vi "MultiPAS-III.vi"() -> ()   [LabVIEW 2011]
uses:
  <vilib>/Analysis/4window.llb/windowTd.ctl
  sub/QMH/QMH Add Message to Queue (Single Element).vi
  sub/QMH/QMH Add Message to Queue (Array).vi
  sub/absCalcPlot_III.vi
  <vilib>/Utility/file.llb/Write To Spreadsheet File (string).vi
  <vilib>/measure/maspectr.llb/FFT Spectrum (Mag-Phase) for 1 Chan.vi
  sub/fftGetMags.vi
  sub/rollingAverage_III.vi
  sub/micUnbundle_III.vi
  <vilib>/Instr/_visa.llb/VISA Configure Serial Port (Instr).vi
  sub/pdNormalize_III.vi
  <vilib>/measure/NI_MAPro.lvlib
  <vilib>/Analysis/NI_AALPro.lvlib
panel:
  out "pd ts (raw)":T1
  out "PAS Save":bool caption="Overtemp"
  in  "Data 2":i32[][](array[numeric])=[[-16374, -7248, 2543, 12030, 20279, 26487, 30037, 30583, 28073, 22744, 15131, 5976, -3818, -13288, -21504, -27663, -31155, -31636, -29064, -23686, -16036, -6862, 2936, 12388, 20571, 26684, 30122, 30546, 27911, 22483, 14793, 5595, -4207, -13644, -21795, -27855, -31232, -31591, -28898, -23423, -15695, -6476, 3323, 12743, 20858, 26873, 30194, 30492, 27744, 22213, 14447, 5207, -4597, -14002, -22082, -28044, -31304, -31540, -28731, -23149, -15348, -6093, 3713, 13101, 21145, 27063, 30265, 30442, 27576, 21943, 14103, 4822, -4984, -14354, -22365, -28230, -31373, -31485, -28556, -22876, -14998, -5702, 4104, 13452, 21428, 27245, 30335, 30388, 27400, 21669, 13754, 4435, -5375, -14705, -22643, -28407, -31436, -31426, -28378, -22598, -14648, -5314, 4497, 13803, 21706, 27423, 30394, 30325, 27221, 21390, 13402, 4045, -5763, -15056, -22921, -28586, -31496, -31361, -28198, -22319, -14297, -4924, 4879, 14151, 21982, 27597, 30451, 30257, 27038, 21107, 13050, 3658, -6149, -15402, -23193, -28754, -31546, -31290, -28010, -22033, -13944, -4536, 5266, 14498, 22252, 27767, 30500, 30184, 26849, 20821, 12696, 3267, -6535, -15748, -23462, -28924, -31596, -31216, -27821, -21748, -13587, -4147, 5653, 14838, 22519, 27930, 30549, 30110, 26658, 20535, 12337, 2878, -6919, -16089, -23727, -29087, -31641, -31137, -27627, -21457, -13229, -3753, 6038, 15181, 22786, 28093, 30591, 30031, 26461, 20243, 11979, 2485, -7303, -16428, -23991, -29244, -31678, -31053, -27426, -21159, -12867, -3360, 6424, 15524, 23043, 28252, 30633, 29946, 26262, 19946, 11617, 2096, -7686, -16764, -24246, -29398, -31712, -30964, -27224, -20862, -12503, -2971, 6803, 15859, 23301, 28401, 30661, 29852, 26058, 19648, 11254, 1703, -8069, -17099, -24500, -29547, -31741, -30870, -27018, -20562, -12138, -2575, 7188, 16192, 23556, 28549, 30689, 29756, 25848, 19348, 10891, 1312, -8448, -17430, -24753, -29691, -31765, -30773, -26806, -20259, -11775, -2186, 7566, 16521, 23801, 28690, 30709, 29656, 25634, 19038, 10523, 919, -8831, -17762, -24997, -29833, -31788, -30672, -26593, -19955, -11409, -1792, 7944, 16850, 24047, 28830, 30724, 29548, 25416, 18729, 10152, 523, -9212, -18092, -25245, -29969, -31805, -30566, -26375, -19647, -11041, -1403, 8319, 17173, 24287, 28963, 30734, 29436, 25192, 18418, 9781, 130, -9587, -18413, -25481, -30101, -31814, -30449, -26150, -19332, -10666, -1007, 8697, 17497, 24524, 29090, 30745, 29325, 24968, 18105, 9408, -263, -9962, -18735, -25718, -30228, -31820, -30334, -25921, -19016, -10296, -618, 9072, 17814, 24756, 29213, 30746, 29202, 24738, 17787, 9036, -657, -10338, -19058, -25951, -30350, -31818, -30214, -25690, -18699, -9922, -224, 9442, 18128, 24984, 29330, 30738, 29078, 24502, 17466, 8658, -1050, -10710, -19371, -26178, -30467, -31814, -30088, -25458, -18382, -9550, 167, 9812, 18440, 25206, 29443, 30732, 28947, 24264, 17143, 8281, -1445, -11083, -19685, -26404, -30581, -31807, -29959, -25221, -18059, -9175, 556, 10178, 18750, 25426, 29548, 30718, 28809, 24018, 16812, 7901, -1842, -11457, -19996, -26624, -30690, -31795, -29824, -24980, -17733, -8799, 950, 10549, 19058, 25643, 29655, 30700, 28673, 23773, 16484, 7523, -2235, -11824, -20304, -26840, -30793, -31772, -29682, -24731, -17402, -8415, 1341, 10916, 19363, 25856, 29755, 30677, 28528, 23522, 16151, 7141, -2626, -12191, -20607, -27051, -30891, -31746, -29536, -24481, -17070, -8035, 1733, 11280, 19664, 26064, 29851, 30648, 28381, 23272, 15818, 6762, -3019, -12555, -20906, -27258, -30984, -31717, -29391, -24226, -16736, -7655, 2128, 11641, 19962, 26270, 29940, 30615, 28229, 23013, 15483, 6376, -3409, -12914, -21204, -27459, -31071, -31684, -29236, -23967, -16398, -7271, 2515, 12005, 20258, 26468, 30024, 30577, 28072, 22753, 15143, 5990, -3802, -13276, -21497, -27660, -31157, -31643, -29076, -23707, -16058, -6886, 2908, 12363, 20550, 26666, 30107, 30536, 27914, 22489, 14805, 5607, -4192, -13633, -21787, -27849, -31230, -31597, -28911, -23438, -15716, -6501, 3298, 12719, 20839, 26858, 30182, 30488, 27744, 22223, 14459, 5225, -4579, -13988, -22071, -28040, -31304, -31549, -28743, -23167, -15368, -6113, 3693, 13076, 21126, 27047, 30255, 30438, 27576, 21950, 14113, 4837, -4971, -14340, -22354, -28224, -31375, -31494, -28570, -22895, -15022, -5725, 4080, 13430, 21408, 27230, 30324, 30384, 27402, 21676, 13766, 4449, -5360, -14694, -22636, -28409, -31440, -31436, -28397, -22617, -14674, -5338, 4467, 13781, 21686, 27408, 30385, 30320, 27224, 21398, 13418, 4062, -5748, -15044, -22913, -28584, -31498, -31368, -28212, -22339, -14321, -4948, 4856, 14131, 21963, 27583, 30440, 30254, 27042, 21118, 13062, 3669, -6137, -15390, -23183, -28751, -31551, -31297, -28024, -22049, -13962, -4556, 5245, 14476, 22235, 27754, 30497, 30186, 26857, 20834, 12710, 3283, -6519, -15733, -23453, -28921, -31600, -31226, -27837, -21765, -13610, -4168, 5628, 14820, 22502, 27918, 30540, 30109, 26664, 20544, 12354, 2891, -6906, -16074, -23719, -29085, -31646, -31148, -27642, -21475, -13251, -3777, 6014, 15160, 22765, 28078, 30583, 30027, 26468, 20251, 11994, 2501, -7292, -16415, -23980, -29242, -31682, -31064, -27443, -21181, -12892, -3386, 6397, 15501, 23026, 28238, 30624, 29944, 26269, 19959, 11633, 2110, -7673, -16753, -24239, -29395, -31719, -30974, -27239, -20882, -12528, -2993, 6782, 15835, 23285, 28390, 30651, 29852, 26063, 19660, 11271, 1720, -8053, -17087, -24493, -29546, -31746, -30880, -27031, -20583, -12163, -2599, 7166, 16173, 23538, 28538, 30684, 29758, 25853, 19356, 10906, 1327, -8433, -17416, -24743, -29688, -31769, -30782, -26821, -20280, -11797, -2208, 7543, 16501, 23786, 28680, 30704, 29656, 25642, 19053, 10540, 936, -8814, -17747, -24989, -29827, -31787, -30678, -26606, -19973, -11430, -1817, 7923, 16829, 24031, 28819, 30721, 29552, 25424, 18746, 10174, 543, -9191, -18072, -25231, -29962, -31802, -30567, -26384, -19660, -11057, -1422, 8302, 17159, 24274, 28952, 30738, 29443, 25205, 18435, 9801, 150, -9568, -18401, -25472, -30095, -31811, -30457, -26163, -19349, -10687, -1031, 8679, 17481, 24511, 29082, 30742, 29327, 24979, 18121, 9431, -241, -9943, -18717, -25707, -30221, -31815, -30337, -25930, -19029, -10312, -631, 9058, 17802, 24745, 29207, 30746, 29209, 24750, 17805, 9057, -634, -10316, -19037, -25937, -30340, -31814, -30217, -25700, -18713, -9939, -240, 9429, 18117, 24976, 29328, 30740, 29088, 24519, 17486, 8682, -1027, -10688, -19352, -26164, -30458, -31810, -30091, -25465, -18390, -9561, 154, 9800, 18433, 25201, 29442, 30735, 28959, 24282, 17165, 8308, -1420, -11063, -19665, -26386, -30570, -31801, -29961, -25227, -18068, -9185, 547, 10171, 18745, 25424, 29552, 30726, 28825, 24038, 16835, 7925, -1815, -11429, -19974, -26608, -30681, -31789, -29826, -24984, -17741, -8807, 938, 10536, 19047, 25636, 29657, 30708, 28685, 23794, 16510, 7550, -2205, -11798, -20280, -26821, -30782, -31766, -29684, -24737, -17411, -8429, 1331, 10906, 19356, 25851, 29758, 30684, 28544, 23546, 16178, 7169, -2598, -12162, -20582, -27035, -30879, -31744, -29540, -24485, -17080, -8048, 1721, 11267, 19655, 26061, 29852, 30654, 28395, 23291, 15843, 6786, -2993, -12527, -20884, -27240, -30974, -31713, -29390, -24230, -16744, -7662, 2115, 11635, 19957, 26268, 29945, 30624, 28246, 23035, 15509, 6406, -3382, -12889, -21180, -27444, -31061, -31677, -29236, -23975, -16408, -7284], [-19329, -1252, 17344, 29341, 30145, 19451, 1353, -17227, -29174, -29920, -19175, -1056, 17506, 29408, 30095, 19300, 1159, -17387, -29238, -29860, -19019, -860, 17671, 29475, 30037, 19143, 960, -17553, -29307, -29809, -18866, -664, 17832, 29545, 29987, 18991, 771, -17707, -29365, -29749, -18707, -466, 17992, 29605, 29926, 18832, 570, -17873, -29434, -29694, -18556, -272, 18151, 29670, 29869, 18676, 375, -18031, -29495, -29633, -18395, -75, 18310, 29729, 29809, 18516, 175, -18194, -29561, -29579, -18238, 120, 18469, 29792, 29750, 18362, -17, -18347, -29617, -29515, -18076, 316, 18629, 29848, 29682, 18197, -218, -18510, -29679, -29456, -17921, 513, 18787, 29910, 29626, 18042, -408, -18664, -29734, -29388, -17757, 709, 18941, 29965, 29560, 17875, -609, -18823, -29791, -29326, -17600, 904, 19095, 30023, 29495, 17717, -802, -18975, -29845, -29260, -17434, 1099, 19251, 30075, 29425, 17551, -1001, -19131, -29901, -29194, -17277, 1296, 19408, 30130, 29359, 17393, -1193, -19284, -29953, -29124, -17112, 1491, 19560, 30184, 29290, 17225, -1392, -19440, -30008, -29056, -16949, 1686, 19713, 30237, 29226, 17069, -1581, -19587, -30054, -28982, -16781, 1883, 19866, 30287, 29151, 16898, -1781, -19742, -30107, -28913, -16616, 2079, 20018, 30337, 29082, 16737, -1973, -19888, -30152, -28838, -16449, 2275, 20167, 30383, 29006, 16564, -2174, -20041, -30200, -28765, -16282, 2471, 20321, 30430, 28934, 16403, -2364, -20187, -30243, -28688, -16113, 2669, 20465, 30470, 28853, 16230, -2568, -20341, -30294, -28618, -15953, 2860, 20615, 30519, 28783, 16070, -2755, -20486, -30335, -28537, -15779, 3057, 20760, 30560, 28700, 15892, -2956, -20637, -30378, -28461, -15613, 3252, 20909, 30605, 28628, 15730, -3145, -20777, -30418, -28377, -15440, 3446, 21054, 30645, 28543, 15557, -3345, -20927, -30460, -28299, -15271, 3643, 21199, 30686, 28465, 15391, -3534, -21066, -30495, -28215, -15100, 3839, 21345, 30722, 28380, 15214, -3734, -21213, -30534, -28134, -14928, 4032, 21487, 30760, 28300, 15044, -3926, -21355, -30570, -28052, -14757, 4225, 21627, 30792, 28209, 14870, -4123, -21501, -30607, -27968, -14586, 4419, 21768, 30832, 28129, 14702, -4314, -21637, -30639, -27880, -14413, 4612, 21907, 30859, 28040, 14521, -4515, -21780, -30675, -27796, -14241, 4804, 22048, 30895, 27953, 14352, -4702, -21919, -30705, -27707, -14064, 4999, 22187, 30922, 27859, 14172, -4900, -22060, -30739, -27620, -13892, 5193, 22326, 30954, 27773, 14003, -5090, -22194, -30765, -27524, -13712, 5386, 22462, 30981, 27679, 13823, -5285, -22333, -30794, -27436, -13538, 5580, 22600, 31013, 27591, 13650, -5476, -22466, -30820, -27343, -13363, 5770, 22732, 31033, 27491, 13468, -5673, -22605, -30848, -27251, -13187, 5964, 22870, 31060, 27401, 13292, -5863, -22736, -30870, -27155, -13010, 6156, 23000, 31079, 27299, 13111, -6058, -22873, -30895, -27060, -12833, 6347, 23134, 31104, 27208, 12936, -6248, -23004, -30918, -26965, -12652, 6536, 23260, 31120, 27106, 12753, -6444, -23136, -30939, -26865, -12472, 6729, 23395, 31148, 27011, 12578, -6634, -23266, -30959, -26766, -12296, 6919, 23523, 31161, 26907, 12392, -6830, -23402, -30982, -26665, -12115, 7109, 23652, 31180, 26809, 12213, -7016, -23524, -30992, -26564, -11932, 7301, 23777, 31195, 26704, 12032, -7210, -23655, -31011, -26464, -11755, 7492, 23907, 31211, 26605, 11855, -7395, -23778, -31024, -26358, -11573, 7680, 24031, 31218, 26494, 11665, -7592, -23908, -31039, -26258, -11392, 7871, 24158, 31237, 26394, 11491, -7775, -24031, -31050, -26153, -11210, 8063, 24281, 31247, 26285, 11302, -7972, -24159, -31062, -26046, -11027, 8250, 24407, 31258, 26180, 11124, -8157, -24276, -31067, -25937, -10841, 8438, 24526, 31265, 26071, 10936, -8347, -24401, -31078, -25829, -10659, 8630, 24649, 31275, 25965, 10755, -8533, -24522, -31087, -25721, -10474, 8816, 24770, 31280, 25853, 10566, -8726, -24641, -31091, -25608, -10290, 9003, 24891, 31287, 25746, 10386, -8910, -24756, -31095, -25498, -10105, 9192, 25008, 31287, 25627, 10196, -9102, -24881, -31101, -25386, -9919, 9381, 25127, 31296, 25521, 10019, -9284, -24994, -31099, -25268, -9732, 9570, 25243, 31293, 25403, 9826, -9476, -25113, -31105, -25157, -9544, 9756, 25359, 31298, 25291, 9645, -9655, -25225, -31099, -25040, -9359, 9942, 25473, 31291, 25167, 9453, -9847, -25341, -31102, -24926, -9173, 10124, 25586, 31294, 25057, 9269, -10029, -25450, -31095, -24809, -8986, 10310, 25696, 31284, 24931, 9078, -10218, -25564, -31094, -24688, -8798, 10497, 25812, 31287, 24819, 8896, -10399, -25673, -31085, -24567, -8608, 10682, 25922, 31278, 24698, 8703, -10587, -25785, -31080, -24448, -8422, 10866, 26033, 31274, 24582, 8522, -10765, -25890, -31067, -24321, -8230, 11050, 26140, 31263, 24455, 8325, -10952, -26001, -31064, -24201, -8040, 11234, 26248, 31255, 24338, 8142, -11132, -26106, -31054, -24079, -7852, 11417, 26353, 31243, 24207, 7948, -11316, -26217, -31041, -23952, -7662, 11601, 26464, 31236, 24089, 7763, -11494, -26315, -31025, -23829, -7471, 11782, 26562, 31217, 23957, 7567, -11682, -26422, -31014, -23702, -7282, 11962, 26667, 31205, 23834, 7383, -11859, -26521, -30998, -23575, -7092, 12144, 26770, 31187, 23704, 7186, -12043, -26626, -30981, -23444, -6900, 12328, 26875, 31176, 23582, 7003, -12218, -26724, -30962, -23316, -6709, 12505, 26971, 31154, 23446, 6805, -12401, -26825, -30946, -23189, -6517, 12687, 27073, 31139, 23322, 6620, -12576, -26919, -30922, -23054, -6323, 12867, 27170, 31114, 23185, 6422, -12760, -27022, -30904, -22923, -6132, 13047, 27272, 31096, 23060, 6237, -12934, -27114, -30879, -22790, -5940, 13222, 27362, 31068, 22921, 6041, -13116, -27212, -30855, -22657, -5748, 13401, 27461, 31048, 22790, 5853, -13289, -27302, -30828, -22522, -5555, 13577, 27549, 31019, 22652, 5652, -13472, -27398, -30806, -22388, -5362, 13753, 27645, 30995, 22521, 5463, -13642, -27487, -30776, -22248, -5169, 13928, 27733, 30963, 22376, 5266, -13823, -27584, -30750, -22113, -4975, 14106, 27828, 30937, 22246, 5082, -13992, -27669, -30717, -21974, -4782, 14280, 27914, 30902, 22101, 4880, -14174, -27760, -30689, -21837, -4588, 14454, 28006, 30875, 21965, 4692, -14340, -27843, -30653, -21693, -4391, 14631, 28092, 30840, 21822, 4494, -14519, -27934, -30620, -21552, -4198, 14805, 28179, 30808, 21688, 4308, -14687, -28015, -30582, -21410, -4004, 14975, 28262, 30770, 21540, 4106, -14861, -28103, -30548, -21268, -3808, 15149, 28349, 30739, 21402, 3916, -15032, -28183, -30512, -21124, -3614, 15319, 28430, 30697, 21255, 3715, -15205, -28267, -30475, -20982, -3421, 15490, 28513, 30664, 21116, 3524, -15376, -28348, -30435, -20837, -3225, 15660, 28592, 30617, 20962, 3327, -15550, -28432, -30397, -20695, -3032, 15829, 28673, 30581, 20820, 3134, -15711, -28506, -30353, -20546, -2837, 15994, 28746, 30530, 20669, 2933, -15887, -28585, -30311, -20400, -2641, 16167, 28828, 30496, 20528, 2745, -16052, -28660, -30264, -20248, -2445, 16335, 28901, 30445, 20376, 2544, -16221, -28737, -30219, -20102, -2250, 16505, 28983, 30406, 20231, 2357, -16381, -28808, -30171, -19950, -2053, 16670, 29053, 30355, 20075, 2154, -16552, -28883, -30127, -19803, -1859, 16835, 29128, 30308, 19930, 1965, -16714, -28952, -30073, -19650, -1663, 17001, 29192, 30255, 19772, 1764, -16881, -29028, -30026, -19496, -1467, 17165, 29268, 30208, 19626, 1572, -17043, -29095, -29977, -19346]]
  out "Filtering":bool caption="Time has Elapsed"
  in  "Switch Filter":bool
  in  "Auto Filter":bool
  out "Elapsed Time (min)":dbl caption="Elapsed Time (s)" format="%#.1g"
  in  "Filter Length (min)":dbl=6.0 caption="Time Target (s)"
  in  "Sample Length (min)":dbl=24.0 caption="Time Target (s)" format="%#.1f"
  out "Time has Elapsed":bool
  in  "Time Target (s)":dbl=1.0
  in  "sweep":bool
  in  "All Emit":bool
  in  "Alignment Mode":bool
  in  "782 Emission":bool
  in  "782 Power (mW)":dbl(slide)=100.0 min=0.0 max=100.0 step=1.0 scale=0.0..100.0
  in  "532 Emission":bool
  in  "532 Power (mW)":dbl(slide)=100.0 min=0.0 max=100.0 step=1.0 scale=0.0..100.0
  in  "423 Power (mW)":dbl(slide)=100.0 min=0.0 max=100.0 step=1.0 scale=0.0..100.0
  in  "423 Emission":bool
  out "Overtemp":bool
  in  "Tab Control":T2(tab)=enum."Frequency Sweep"
  out "sweeps":path caption="Microphone File Path"
  in  "save interval (ms)":u32=1000
  out "Error Console":T3
  out "pas":path caption="Microphone File Path"
  out "Laser Temperatures":T4(graph)
  in  "pd id":u32=1
  in  "mic id":u32
  in  "mic cal, scu":dbl=5.41531278804282e-05 format="%#_3e"
  in  "mic cal, scu":dbl=5.59307241877627e-05 format="%#_3e"
  in  "423 Port":refnum<visa-resource-name>="COM4"
  in  "532 Port":refnum<visa-resource-name>="COM5"
  in  "782 Port":refnum<visa-resource-name>="COM6"
  in  "Teensy Port":refnum<visa-resource-name>="COM3"
  in  "Save Data":bool
  in  "405 PD Cal 3":dbl=0.039
  in  "532 PD Cal 3":dbl=0.027
  in  "660 PD Cal 3":dbl=0.024
  out "freqscan":cluster{i32[], "Best Gaussian Fit":dbl[]}[](graph) caption="Frequency Sweep"
  out "sweep progress":dbl(slide) scale=0.0..1.0
  in  "Autosweep?":bool=TRUE
  in  "set freqs":bool
  out "Calculated Resonance (Hz)":dbl=1370.0
  in  "Data Start Frequency (Hz)":i32=1355
  in  "Data End Frequency (Hz)":i32=1405
  in  "423 F (Hz)":i32=1368
  in  "532 F (Hz)":i32=1372
  in  "782 F (Hz)":i32=1370
  in  "Chart Rolling Average":i32=16
  out "pdwave":waveform(i32)(graph) caption="Photodiode Waveform"
  out "pd ts":cluster{dbl, dbl, dbl}(graph)
  out "pdfft":cluster{"f0":dbl, "df":dbl, "magnitude":dbl[]}(graph) caption="Photodiode FFT"
  in  "rollavg":i32=16 caption="Dispaly Averaging (Transfers to Absorption Data!)"
  out "mic ts":T5(graph)
  out "micfft":cluster{"f0":dbl, "df":dbl, "magnitude":dbl[]}(graph) caption="Photodiode FFT"
  out "micwave":waveform(i32)(graph) caption="Photodiode Waveform"
  in  "getbkg":bool
  out "AAE":dbl(graph)
  in  "Bkg Values (mV)":cluster{dbl, dbl, dbl}
  out "Absorption Spectrum":cluster{dbl[], "Best Power Fit":dbl[]}[](graph)
  out "abs ts":cluster{dbl, dbl, dbl}(graph)
  in  "cellcal":dbl=95000.0 caption="Cell Calibration Coefficient (mV/mW)"
  out "Status":string
  in  "Exit":bool
  in  "State Variables":cluster{"CurrentFile":path}
  # "MultiPAS-III | AeroSmith Labs (2017)"
  # "Laser Control"
  # "Filter Control"
  # "Communications"
  # "Sound Card Parameters"
  # "Data File Options"
  # "File paths are populated automatically at <...\\My Documents\\MultiPAS Data\\>.  To save in another location, turn on \"Save Data\" and follow the prompts to choose an alternate working directory."
  # "Photodiode Calibration"
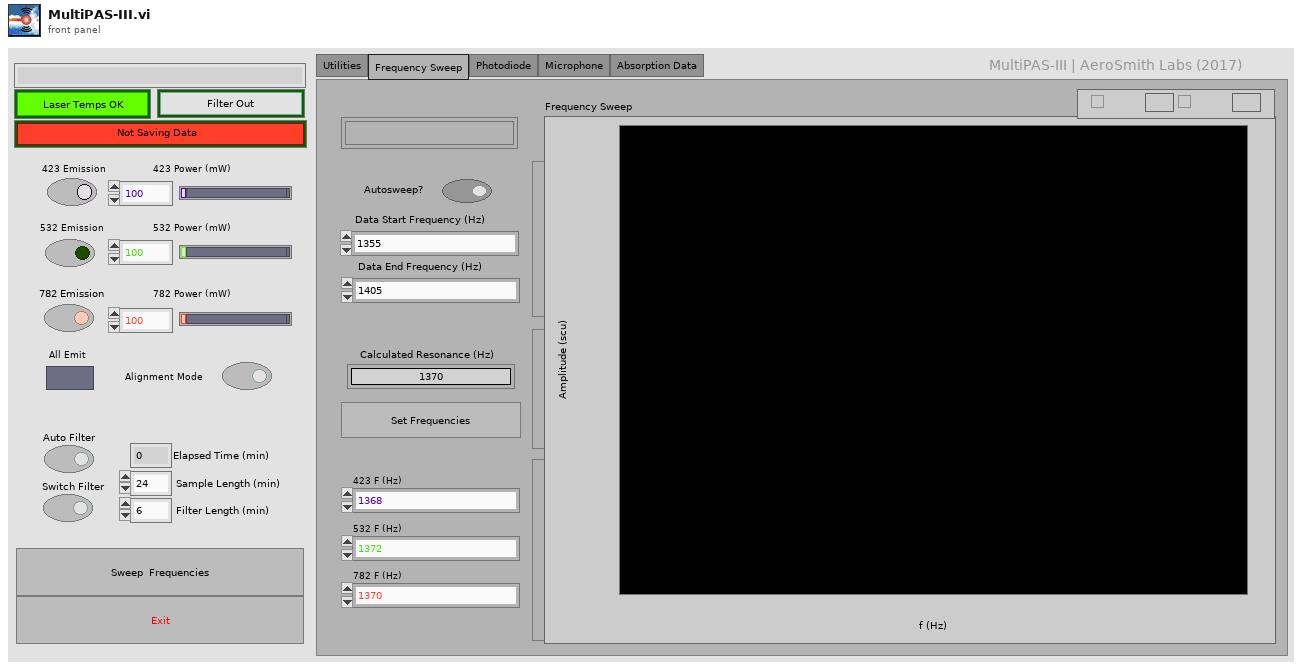
[diagram p1: front panel]
types:
  T1 = cluster{"405 Mean":dbl, "532 Mean":dbl, "660 Mean":dbl}
  T2 = enum32{"Utilities", "Frequency Sweep", "Photodiode", "Microphone", "Absorption Data"}
  T3 = cluster{"status":bool, "code":i32, "Message":string}
  T4 = cluster{"Temp (C)":dbl, "Temp (C)":dbl, "Temp (C)":dbl}
  T5 = cluster{"422 Mean":dbl, "532 Mean":dbl, "785 Mean":dbl}
  T6 = cluster{"# buffers":i32, "Buffer size":i32, "unit (ms)":enum16{"time (ms)", "Samples"}}
  T7 = typedef "SoundHandle.ctl" = cluster{"DeviceID":u16, "Samples/buf":u32, "Sampl rate":u32, "Bits/sample":u16, "Channels":u8, "Opened":bool}
  T8 = typedef "NI_AALPro.lvlib/windowTd.ctl" = u32
  T9 = cluster{"785 New Array":dbl[], "785 Mean":dbl, "785 SD":dbl}
  T10 = cluster{"532 New Array":dbl[], "532 Mean":dbl, "532 SD":dbl}
  T11 = cluster{"422 New Array":dbl[], "422 Mean":dbl, "422 SD":dbl}
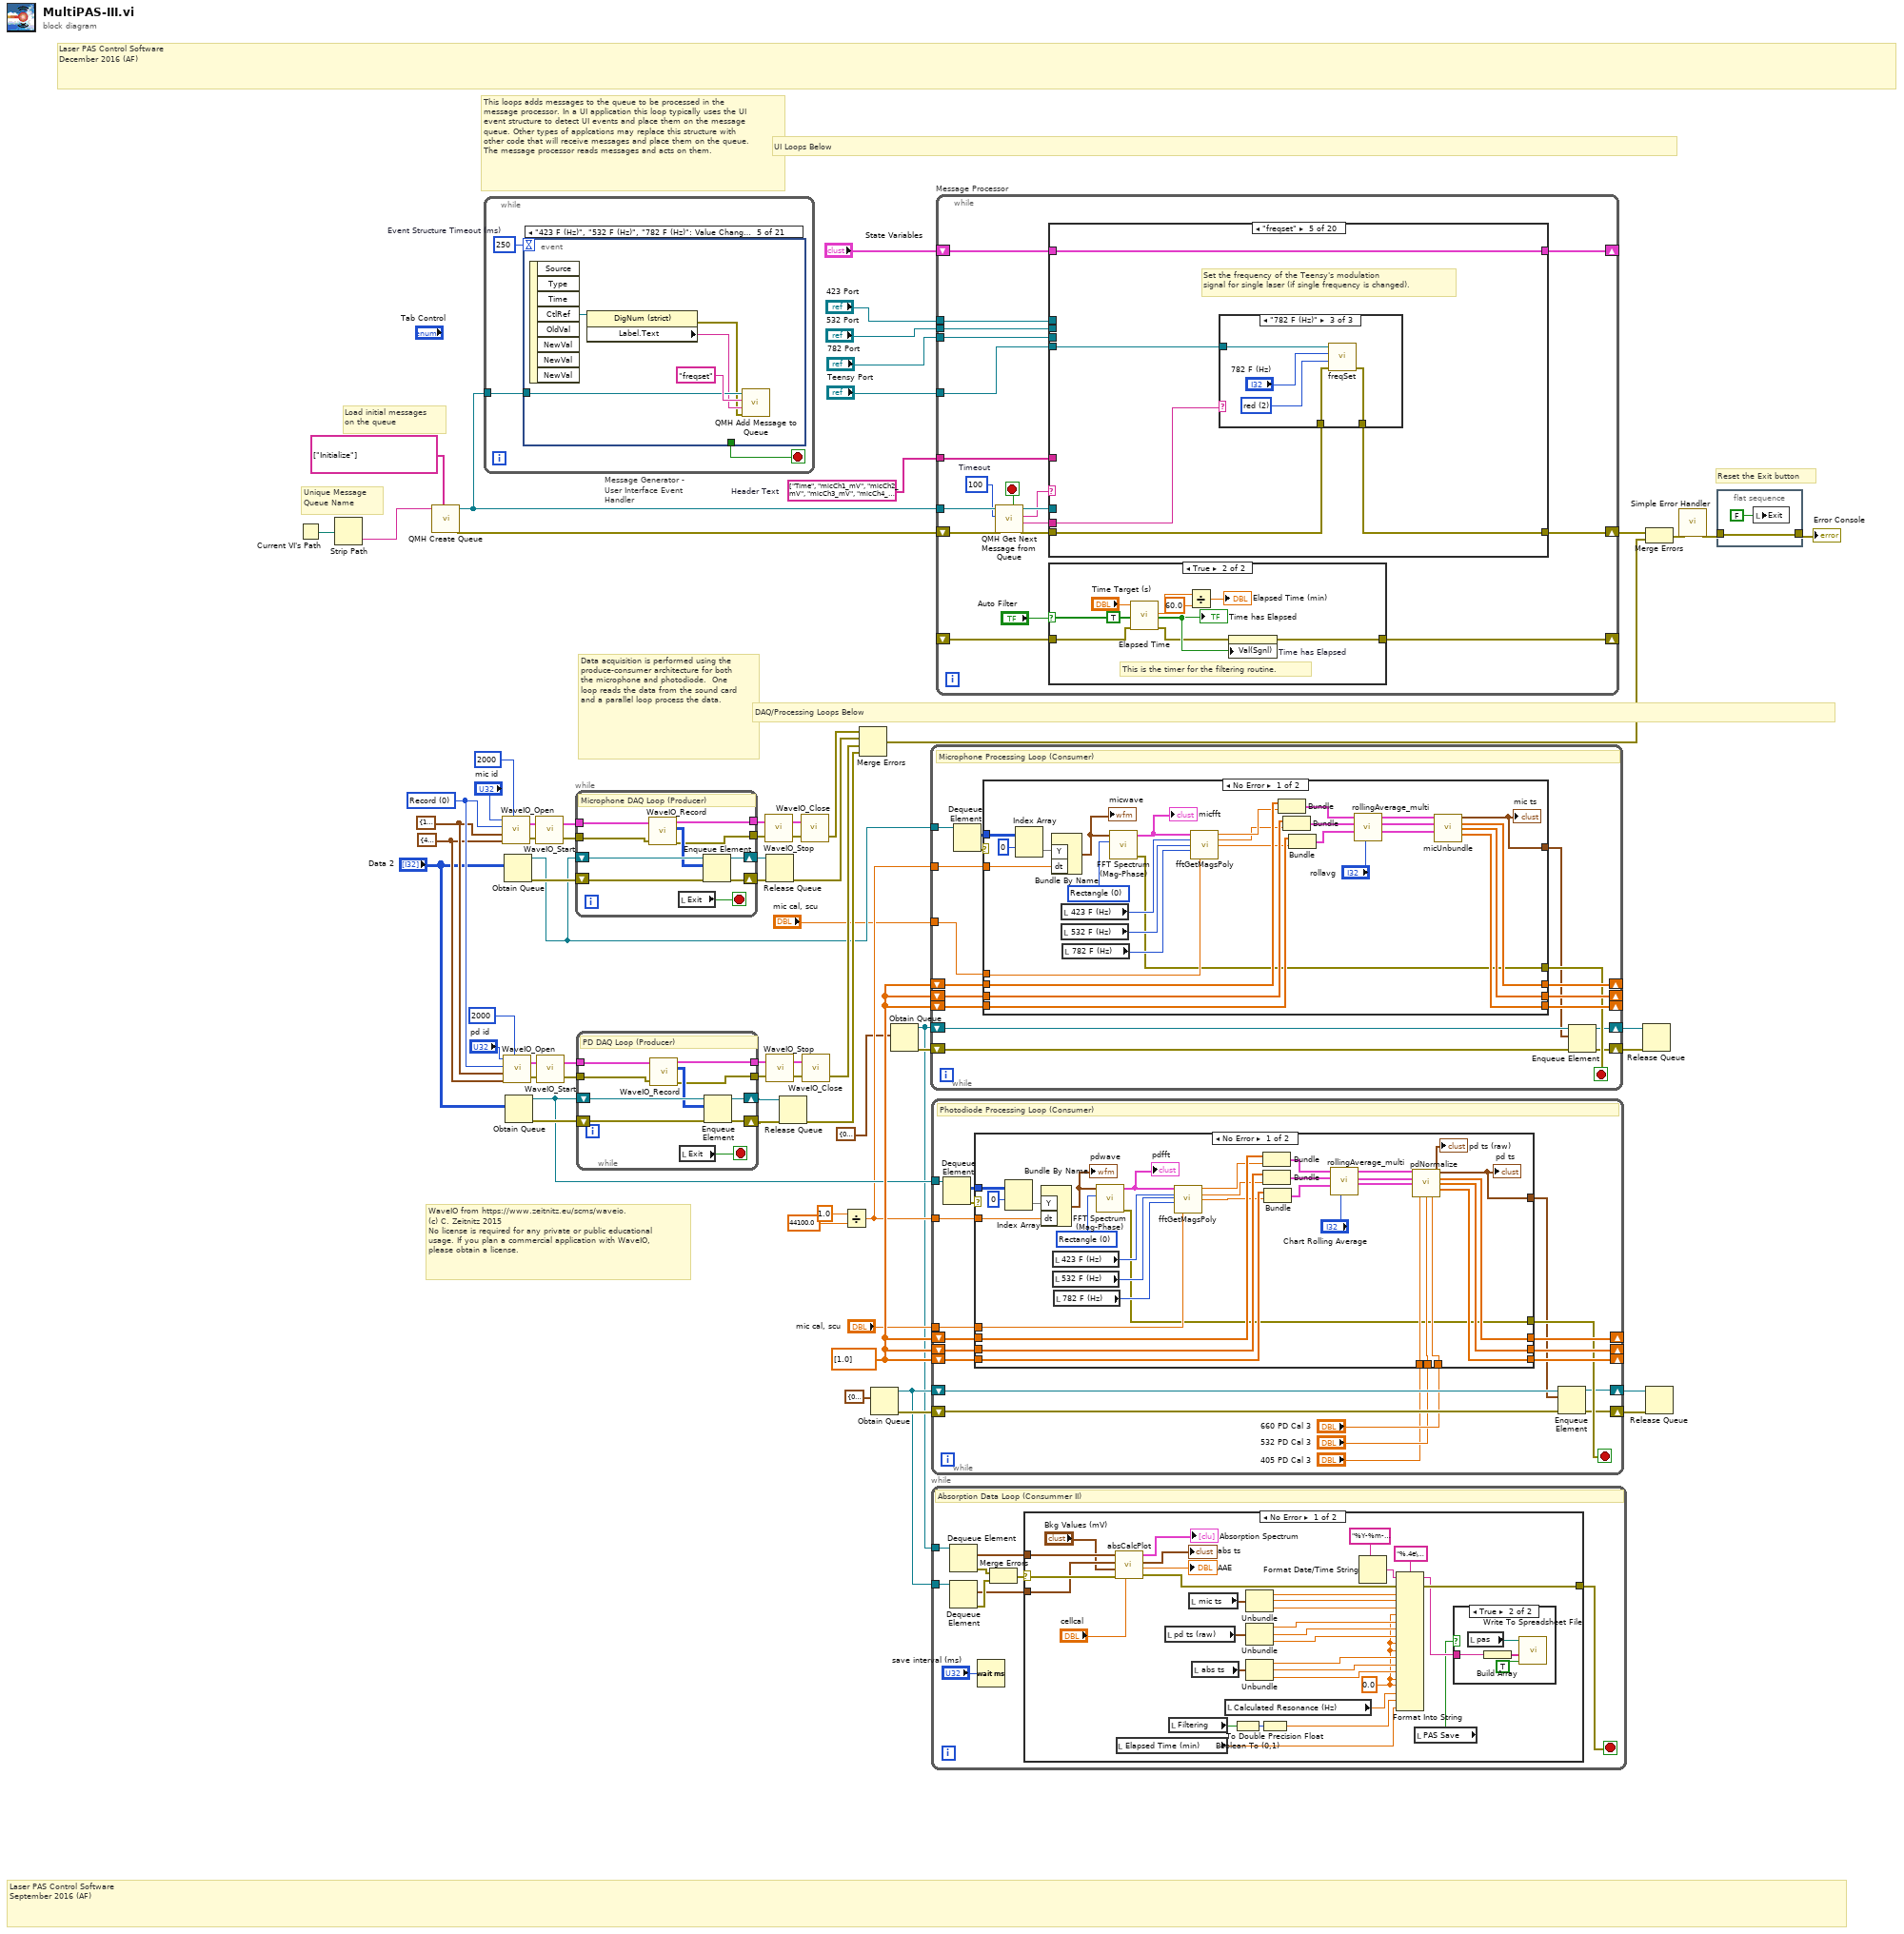
[diagram p0: block diagram]
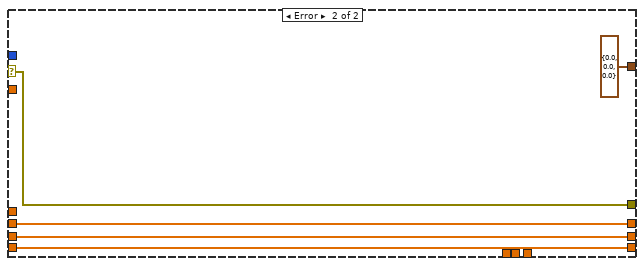
[diagram p4: hidden frame]
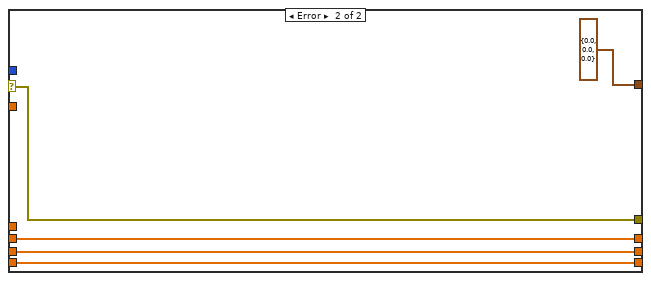
[diagram p5: hidden frame]
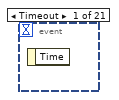
[diagram p6: hidden frame]
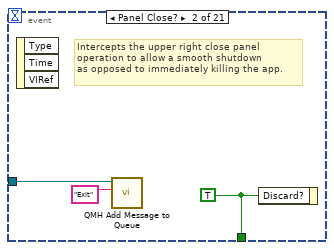
[diagram p7: hidden frame]
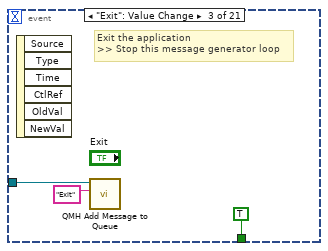
[diagram p8: hidden frame]
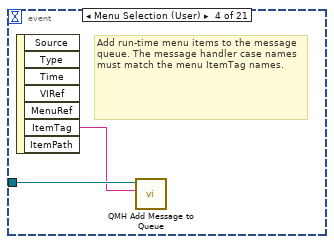
[diagram p9: hidden frame]
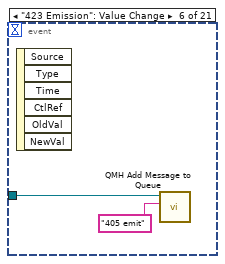
[diagram p10: hidden frame]
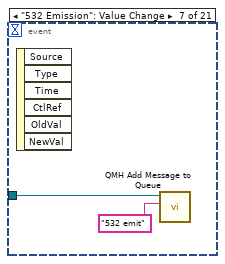
[diagram p11: hidden frame]
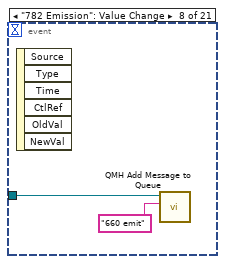
[diagram p12: hidden frame]
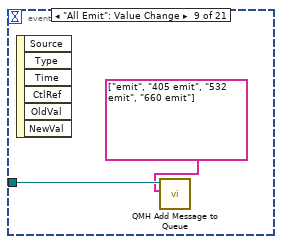
[diagram p13: hidden frame]
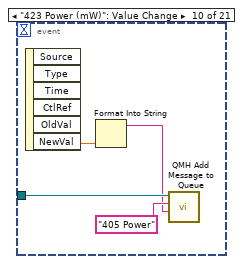
[diagram p14: hidden frame]
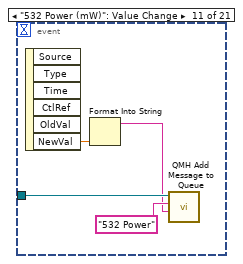
[diagram p15: hidden frame]
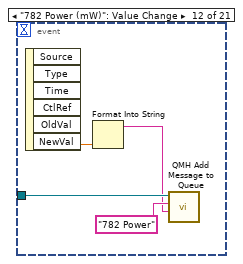
[diagram p16: hidden frame]
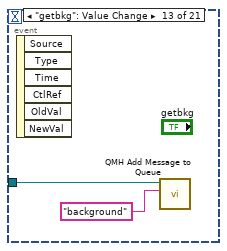
[diagram p17: hidden frame]
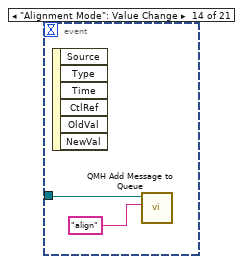
[diagram p18: hidden frame]
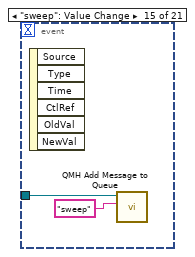
[diagram p19: hidden frame]
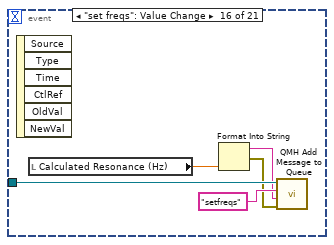
[diagram p20: hidden frame]
diagram:
  w1 = string[] ["Time", "micCh1_mV", "micCh2_mV", "micCh3_mV", "micCh4_mV", "pdCh1_mV", "pdCh2_mV", "pdCh3_mV", "pdCh4_mV", "tau_sec", "babsCh1_Mm", "babsCh2_Mm", "babsCh3_Mm", "babsCh4_Mm", "bext_Mm", "fres_Hz", "filter_state", "elapsedTime_min"]  # Header Text
  w21 = T6 {"# buffers"=10, "Buffer size"=44100, "unit (ms)"=enum."Samples"} ("Buffer")
  w20 = cluster{"Rate":i32, "Bits":i32, "Channels":i32} {"Rate"=44100, "Bits"=24, "Channels"=2} ("Format")
  w22 = u16 0 items=["Record", "Play", "Loopback", "ASIO input", "ASIO output"] ("Direction (Record)")
  w52 = dbl[] [1.0] ("X")
  # "Laser PAS Control Software\nSeptember 2016 (AF)"
  # "Laser PAS Control Software\nDecember 2016 (AF)"
  # "Data acquisition is performed using the produce-consumer architecture for both the microphone and photodiode.  One loop reads the data from the sound card and a parallel loop process the data."
  # "WaveIO from https://www.zeitnitz.eu/scms/waveio.\n(c) C. Zeitnitz 2015\nNo license is required for any private or public educational usage. If you plan a commercial application with WaveIO, please obtain a license."
  # "This loops adds messages to the queue to be processed in the message processor. In a UI application this loop typically uses the UI event structure to detect UI events and place them on the message queue. Other types of applcations may replace this structure with other code that will receive messages and place them on the queue.  The message processor reads messages and acts on them."
  # "Reset the Exit button"
  # "Unique Message\nQueue Name"
  # "Load initial messages\non the queue"
  # "DAQ/Processing Loops Below"
  # "UI Loops Below"
  n1 = Current VI's Path() -> (path=w67:path)
  n2 = Strip Path(path=w67) -> (name=w68:string)  [unwired: 1 out]
  n3 = call "QMH Create Queue.vi"("Initial Messages"=string[] ["Initialize"], "Message queue name (unnamed)"=w68) -> ("error out"=w64:errorcluster, "queue out"=w49:refnum<queue>)  [unwired: 8 in]
  n4 = while "Message Generator - User Interface Event Handler" {
    tunnel: w49 -> [w69]
    stop <- w70 stop-if-true
    w71 = 250  # Event Structure Timeout (ms)
    n5 = event shown="[4] \"423 F (Hz)\", \"532 F (Hz)\", \"782 F (Hz)\": Value Change" {
      selector: _ -> [_ _ _ _ _ _ _ _ _ _ _ _ _ _ _ _ _ _ _ _ _]
      dyn-events: _ -> [_ _ _ _ _ _ _ _ _ _ _ _ _ _ _ _ _ _ _ _ _]
      timeout: w71 -> [_ _ _ _ _ _ _ _ _ _ _ _ _ _ _ _ _ _ _ _ _]
      tunnel: [_ w74 TRUE ("Discard?") _ _ _ _ _ _ _ _ _ _ _ _ _ _ _ _ _ _] -> w70
      tunnel: w69 -> [_ w73 w76 w79 w83 w85 w87 w89 w92 w95 w99 w103 w105 w107 w110 w114 w119 w124 w128 w133 w135]
      event Timeout {
        n6 = event-data() -> ()  [unwired: 1 in, 1 out]
      }
      event Panel Close? {
        w74 = TRUE ("Discard?")
        # "Intercepts the upper right close panel\noperation to allow a smooth shutdown\nas opposed to immediately killing the app."
        n7 = event-data() -> ()  [unwired: 1 in, 3 out]
        n8 = call-poly "QMH Add Message to Queue.vi"("Message"="Exit", "queue in"=w73) -> ()  [unwired: 8 in, 2 out]
        n9 = event-data("Discard?"=w74) -> ()  [unwired: 1 in, 1 out]
      }
      event "Exit": Value Change {
        # "Exit the application\n>> Stop this message generator loop"
        n10 = event-data() -> ()  [unwired: 1 in, 6 out]
        n11 = call-poly "QMH Add Message to Queue.vi"("Message"="Exit", "queue in"=w76) -> ()  [unwired: 8 in, 2 out]
      }
      event Menu Selection (User) {
        # "Add run-time menu items to the message\nqueue. The message handler case names must match the menu ItemTag names."
        n12 = event-data() -> ("ItemTag"=w78:string)  [unwired: 1 in, 6 out]
        n13 = call-poly "QMH Add Message to Queue.vi"("Message"=w78, "queue in"=w79) -> ()  [unwired: 8 in, 2 out]
      }
      event "423 F (Hz)", "532 F (Hz)", "782 F (Hz)": Value Change {
        n14 = event-data() -> ("CtlRef"=w82:refnum<vi>)  [unwired: 1 in, 7 out]
        n15 = property class="DigNum (strict)"(reference=w82) -> (error out=w80:errorcluster, "Label.Text"=w81:string)  [unwired: 1 in, 1 out]
        n16 = call-poly "QMH Add Message to Queue.vi"("error in (no error)"=w80, "Parameter"=w81, "Message"="freqset", "queue in"=w83) -> ()  [unwired: 6 in, 2 out]
      }
      event "423 Emission": Value Change {
        n17 = event-data() -> ()  [unwired: 1 in, 6 out]
        n18 = call-poly "QMH Add Message to Queue.vi"("Message"="405 emit", "queue in"=w85) -> ()  [unwired: 8 in, 2 out]
      }
      event "532 Emission": Value Change {
        n19 = event-data() -> ()  [unwired: 1 in, 6 out]
        n20 = call-poly "QMH Add Message to Queue.vi"("Message"="532 emit", "queue in"=w87) -> ()  [unwired: 8 in, 2 out]
      }
      event "782 Emission": Value Change {
        n21 = event-data() -> ()  [unwired: 1 in, 6 out]
        n22 = call-poly "QMH Add Message to Queue.vi"("Message"="660 emit", "queue in"=w89) -> ()  [unwired: 8 in, 2 out]
      }
      event "All Emit": Value Change {
        n23 = event-data() -> ()  [unwired: 1 in, 6 out]
        n24 = call-poly "QMH Add Message to Queue.vi"("Messages"=string[] ["emit", "405 emit", "532 emit", "660 emit"], "queue in"=w92) -> ()  [unwired: 8 in, 2 out]
      }
      event "423 Power (mW)": Value Change {
        n25 = event-data() -> ("NewVal"=w94:dbl)  [unwired: 1 in, 5 out]
        n26 = Format Into String(w94) -> (resulting string=w93:string)  [unwired: 3 in, 1 out]
        n27 = call-poly "QMH Add Message to Queue.vi"("Parameter"=w93, "Message"="405 Power", "queue in"=w95) -> ()  [unwired: 7 in, 2 out]
      }
      event "532 Power (mW)": Value Change {
        n28 = event-data() -> ("NewVal"=w98:dbl)  [unwired: 1 in, 5 out]
        n29 = Format Into String(w98) -> (resulting string=w97:string)  [unwired: 3 in, 1 out]
        n30 = call-poly "QMH Add Message to Queue.vi"("Parameter"=w97, "Message"="532 Power", "queue in"=w99) -> ()  [unwired: 7 in, 2 out]
      }
      event "782 Power (mW)": Value Change {
        n31 = event-data() -> ("NewVal"=w102:dbl)  [unwired: 1 in, 5 out]
        n32 = Format Into String(w102) -> (resulting string=w101:string)  [unwired: 3 in, 1 out]
        n33 = call-poly "QMH Add Message to Queue.vi"("Parameter"=w101, "Message"="782 Power", "queue in"=w103) -> ()  [unwired: 7 in, 2 out]
      }
      event "getbkg": Value Change {
        n34 = event-data() -> ()  [unwired: 1 in, 6 out]
        n35 = call-poly "QMH Add Message to Queue.vi"("Message"="background", "queue in"=w105) -> ()  [unwired: 8 in, 2 out]
      }
      event "Alignment Mode": Value Change {
        n36 = event-data() -> ()  [unwired: 1 in, 6 out]
        n37 = call-poly "QMH Add Message to Queue.vi"("Message"="align", "queue in"=w107) -> ()  [unwired: 8 in, 2 out]
      }
      event "sweep": Value Change {
        n38 = event-data() -> ()  [unwired: 1 in, 6 out]
        n39 = call-poly "QMH Add Message to Queue.vi"("Message"="sweep", "queue in"=w110) -> ()  [unwired: 8 in, 2 out]
      }
      event "set freqs": Value Change {
        n40 = event-data() -> ()  [unwired: 1 in, 6 out]
        n41 = local read "Calculated Resonance (Hz)"() -> (w113:dbl)
        n42 = Format Into String(w113) -> (resulting string=w112:string, error out=w111:errorcluster)  [unwired: 3 in]
        n43 = call-poly "QMH Add Message to Queue.vi"("error in (no error)"=w111, "Parameter"=w112, "Message"="setfreqs", "queue in"=w114) -> ()  [unwired: 6 in, 2 out]
      }
      event "Save Data": Value Change {
        n44 = event-data() -> ("NewVal"=w118:bool)  [unwired: 1 in, 5 out]
        n45 = Format Into String(w118) -> (resulting string=w117:string, error out=w116:errorcluster)  [unwired: 3 in]
        n46 = call-poly "QMH Add Message to Queue.vi"("error in (no error)"=w116, "Parameter"=w117, "Message"="namefiles", "queue in"=w119) -> ()  [unwired: 6 in, 2 out]
      }
      event "Switch Filter": Value Change {
        n47 = event-data() -> ("NewVal"=w123:bool)  [unwired: 1 in, 5 out]
        n48 = local write "Filtering"(w123) -> ()
        n49 = Format Into String(w123) -> (resulting string=w121:string)  [unwired: 3 in, 1 out]
        n50 = call-poly "QMH Add Message to Queue.vi"("Parameter"=w121, "Message"="filterswitch", "queue in"=w124) -> ()  [unwired: 7 in, 2 out]
      }
      event "Time has Elapsed": Value Change {
        n51 = event-data() -> ("NewVal"=w127:bool)  [unwired: 1 in, 5 out]
        n52 = local read "Filtering"() -> (w126:bool)
        n53 = call "filterCreateMsg.vi"("time elapsed?"=w127, "auto sweep (true)"="Autosweep?", "filtering (true)"=w126, "queue in"=w128) -> ()  [unwired: 6 in, 2 out]
      }
      event "Calculated Resonance (Hz)": Value Change {
        n54 = event-data() -> ("NewVal"=w131:dbl)  [unwired: 1 in, 5 out]
        n55 = Format Into String(w131) -> (resulting string=w129:string, error out=w130:errorcluster)  [unwired: 3 in]
        n56 = call-poly "QMH Add Message to Queue.vi"("error in (no error)"=w130, "Parameter"=w129, "Message"="setfreqs", "queue in"=w133) -> ()  [unwired: 6 in, 2 out]
      }
      event "PAS Save": Value Change {
        n57 = event-data() -> ()  [unwired: 1 in, 6 out]
        n58 = call-poly "QMH Add Message to Queue.vi"("Message"="setwd", "queue in"=w135) -> ()  [unwired: 8 in, 2 out]
      }
    }
  }
  n59 = call <userlib>:"WaveIO_Open.vi"("Watchdog timeout (msec) (default=OFF)"=2000, "Format (44kHz, 16Bit, stereo)"=w20, "Buffer Config"=w21, "Direction (Record)"=w22, "idev"="mic id") -> ("error out"=w45:errorcluster, "Sound Handle Out"=w46:T7)  [unwired: 1 in]
  n60 = call <userlib>:"WaveIO_Open.vi"("Watchdog timeout (msec) (default=OFF)"=2000, "Format (44kHz, 16Bit, stereo)"=w20, "Buffer Config"=w21, "Direction (Record)"=w22, "idev"="pd id") -> ("error out"=w31:errorcluster, "Sound Handle Out"=w30:T7)  [unwired: 1 in]
  n61 = Obtain Queue(element data type="Data 2") -> (queue out=w14:refnum<queue>, error out=w53:errorcluster)  [unwired: 4 in, 1 out]
  n62 = Obtain Queue(element data type="Data 2") -> (queue out=w18:refnum<queue>, error out=w27:errorcluster)  [unwired: 4 in, 1 out]
  n63 = call <userlib>:"WaveIO_Start.vi"("error in (no error)"=w45, "Handle"=w46) -> ("error out"=w43:errorcluster, "Handle Out"=w44:T7)
  n64 = call <userlib>:"WaveIO_Start.vi"("error in (no error)"=w31, "Handle"=w30) -> ("error out"=w33:errorcluster, "Handle Out"=w32:T7)
  n65 = while {
    shift-right: [w144] -> w54
    shift-left: w14 -> [w142]
    shift-right: [w145] -> w55
    shift-left: w53 -> [w143]
    tunnel: w44 -> [w140]
    tunnel: w43 -> [w139]
    tunnel: [w137] -> w40
    tunnel: [w136] -> w39
    stop <- w141 stop-if-true
    # "Microphone DAQ Loop (Producer)"
    n66 = call <userlib>:"WaveIO_Record.vi"("Handle"=w140, "error in (no error)"=w139) -> ("Handle Out"=w137:T7, "Data"=w138:i32[][], "error out"=w136:errorcluster)  [unwired: 1 in, 2 out]
    n67 = local read "Exit"() -> (w141:bool)
    n68 = Enqueue Element(queue=w142, element=w138, error in (no error)=w143) -> (queue out=w144:refnum<queue>, error out=w145:errorcluster)  [unwired: 1 in, 1 out]
  }
  n69 = while {
    shift-right: [w154] -> w26
    shift-left: w18 -> [w152]
    shift-right: [w155] -> w25
    shift-left: w27 -> [w153]
    tunnel: w32 -> [w150]
    tunnel: w33 -> [w149]
    tunnel: [w147] -> w36
    tunnel: [w146] -> w37
    stop <- w151 stop-if-true
    # "PD DAQ Loop (Producer)"
    n70 = call <userlib>:"WaveIO_Record.vi"("Handle"=w150, "error in (no error)"=w149) -> ("Handle Out"=w147:T7, "Data"=w148:i32[][], "error out"=w146:errorcluster)  [unwired: 1 in, 2 out]
    n71 = local read "Exit"() -> (w151:bool)
    n72 = Enqueue Element(queue=w152, element=w148, error in (no error)=w153) -> (queue out=w154:refnum<queue>, error out=w155:errorcluster)  [unwired: 1 in, 1 out]
  }
  n73 = call <userlib>:"WaveIO_Stop.vi"("error in (no error)"=w39, "Handle"=w40) -> ("error out"=w41:errorcluster, "Handle Out"=w42:T7)
  n74 = Release Queue(queue=w54, error in (no error)=w55) -> (error out=w51:errorcluster)  [unwired: 1 in, 2 out]
  n75 = call <userlib>:"WaveIO_Stop.vi"("error in (no error)"=w37, "Handle"=w36) -> ("error out"=w35:errorcluster, "Handle Out"=w34:T7)
  n76 = Release Queue(queue=w26, error in (no error)=w25) -> (error out=w24:errorcluster)  [unwired: 1 in, 2 out]
  n77 = call <userlib>:"WaveIO_Close.vi"("error in (no error)"=w41, "Handle"=w42) -> ("error out"=w38:errorcluster)  [unwired: 1 out]
  n78 = call <userlib>:"WaveIO_Close.vi"("error in (no error)"=w35, "Handle"=w34) -> ("error out"=w23:errorcluster)  [unwired: 1 out]
  n79 = Divide(x=1.0, y=44100.0) -> (x/y=w15:dbl)
  n80 = Merge Errors(w38, w51, w23, w24) -> (w50:errorcluster)
  n81 = Obtain Queue(element data type=cluster{dbl, dbl, dbl} {0.0, 0.0, 0.0}) -> (queue out=w3:refnum<queue>, error out=w8:errorcluster)  [unwired: 4 in, 1 out]
  n82 = Obtain Queue(element data type=cluster{dbl, dbl, dbl} {0.0, 0.0, 0.0}) -> (queue out=w2:refnum<queue>, error out=w11:errorcluster)  [unwired: 4 in, 1 out]
  n83 = while {
    tunnel: w14 -> [w172]
    shift-right: [w169] -> _
    shift-left: w52 -> [w166]
    shift-right: [w168] -> _
    shift-left: w52 -> [w165]
    shift-right: [w167] -> _
    shift-left: w52 -> [w164]
    tunnel: w15 -> [w162]
    tunnel: "mic cal, scu" -> [w161]
    shift-right: [w159] -> w10
    shift-left: w2 -> [w158]
    shift-right: [w156] -> w9
    shift-left: w11 -> [w160]
    stop <- w163 stop-if-true
    # "Microphone Processing Loop (Consumer)"
    n84 = Dequeue Element(queue=w172) -> (element=w170:i32[][], error out=w171:errorcluster)  [unwired: 2 in, 2 out]
    n85 = case shown="No Error" w171 {
      selector: w171 -> [_ w203]
      tunnel: w170 -> [w196 _]
      tunnel: w166 -> [w200 w206]
      tunnel: w165 -> [w199 w204]
      tunnel: w164 -> [w198 w205]
      tunnel: [w176 w206] -> w169
      tunnel: [w175 w204] -> w168
      tunnel: [w174 w205] -> w167
      tunnel: [w173 w203] -> w163
      tunnel: w162 -> [w194 _]
      tunnel: w161 -> [w188 _]
      tunnel: [w177 T1 {"405 Mean"=0.0, "532 Mean"=0.0, "660 Mean"=0.0}] -> w157
      frame No Error {
        w201 = T8 0 items=["Rectangle"=0, "Hanning"=1, "Hamming"=2, "Blackman-Harris"=3, "Exact Blackman"=4, "Blackman"=5, "Flat Top"=6, "4 Term B-Harris "=7, "7 Term B-Harris"=8, "Low Sidelobe"=9, "Blackman Nuttall"=11, "Triangle"=30, "Bartlett-Hanning"=31, "Bohman"=32, "Parzen"=33, "Welch"=34, "Kaiser"=60, "Dolph-Chebyshev"=61, "Gaussian"=62] ("window")
        n86 = Index Array(array=w196, index (row)=0) -> (element=w195:i32[])  [unwired: 1 in]
        n87 = Bundle By Name("Y"=w195, "dt"=w194) -> (w193:waveform(i32))  [unwired: 1 in]
        "micwave" <- w193
        n88 = local read "423 F (Hz)"() -> (w191:i32)
        n89 = local read "532 F (Hz)"() -> (w190:i32)
        n90 = local read "782 F (Hz)"() -> (w189:i32)
        n91 = call-poly <vilib>:"FFT Spectrum (Mag-Phase).vi"("window"=w201, "time signal"=w193) -> ("error out"=w173:errorcluster, "magnitude"=w192:cluster{"f0":dbl, "df":dbl, "magnitude":dbl[]})  [unwired: 5 in, 3 out]
        "micfft" <- w192
        n92 = call-poly "fftGetMagsPoly.vi"("input cluster"=w192, "422 F (Hz)"=w191, "532 F (Hz)"=w190, "785 F (Hz)"=w189, "unit cal, scu"=w188) -> ("mag422 (mV)"=w183:dbl, "mag532 (mV)"=w182:dbl, "mag785 (mV)"=w181:dbl)  [unwired: 8 in]
        n93 = Bundle("X"=w200, "mag422 (mV)"=w183) -> (w187:cluster{"X":dbl[], "mag422 (mV) ":dbl})  [unwired: 1 in]
        n94 = Bundle("X"=w199, "mag532 (mV)"=w182) -> (w186:cluster{"X":dbl[], "mag532 (mV)":dbl})  [unwired: 1 in]
        n95 = Bundle("X"=w198, "mag785 (mV)"=w181) -> (w185:cluster{"X":dbl[], "mag785 (mV)":dbl})  [unwired: 1 in]
        n96 = call-poly "rollingAverage_multi.vi"("Magnitude Averaging (no. Avgs.)"="rollavg", "785nm"=w185, "532nm"=w186, "422nm"=w187) -> ("785nm Data"=w178:T9, "532nm Data"=w179:T10, "422nm Data"=w180:T11)  [unwired: 5 in]
        n97 = call-poly "micUnbundle.vi"("422nm Data"=w180, "532nm Data"=w179, "785nm Data"=w178) -> ("Output Cluster"=w177:T5, "422 New Array"=w176:dbl[], "532 New Array"=w175:dbl[], "785 New Array"=w174:dbl[])  [unwired: 9 in]
        "mic ts" <- w177
      }
      frame Error {
      }
    }
    n98 = Enqueue Element(queue=w158, element=w157, error in (no error)=w160) -> (queue out=w159:refnum<queue>, error out=w156:errorcluster)  [unwired: 1 in, 1 out]
  }
  n99 = while {
    shift-right: [w224] -> _
    shift-left: w52 -> [w221]
    shift-right: [w223] -> _
    shift-left: w52 -> [w220]
    shift-right: [w222] -> _
    shift-left: w52 -> [w219]
    tunnel: w18 -> [w217]
    tunnel: w15 -> [w216]
    tunnel: "mic cal, scu" -> [w215]
    shift-right: [w212] -> w7
    shift-left: w3 -> [w213]
    shift-right: [w211] -> w6
    shift-left: w8 -> [w214]
    stop <- w218 stop-if-true
    # "Photodiode Processing Loop (Consumer)"
    n100 = Dequeue Element(queue=w217) -> (element=w225:i32[][], error out=w226:errorcluster)  [unwired: 2 in, 2 out]
    n101 = case shown="No Error" w226 {
      selector: w226 -> [_ w261]
      tunnel: w225 -> [w254 _]
      tunnel: w221 -> [w258 w264]
      tunnel: w220 -> [w257 w262]
      tunnel: w219 -> [w256 w263]
      tunnel: [w234 w264] -> w224
      tunnel: [w233 w262] -> w223
      tunnel: [w232 w263] -> w222
      tunnel: [w228 w261] -> w218
      tunnel: w216 -> [w252 _]
      tunnel: w215 -> [w246 _]
      tunnel: "660 PD Cal 3" -> [w229 _]
      tunnel: "532 PD Cal 3" -> [w230 _]
      tunnel: "405 PD Cal 3" -> [w231 _]
      tunnel: [w235 cluster{dbl, dbl, dbl} {0.0, 0.0, 0.0}] -> w210
      frame No Error {
        w259 = T8 0 items=["Rectangle"=0, "Hanning"=1, "Hamming"=2, "Blackman-Harris"=3, "Exact Blackman"=4, "Blackman"=5, "Flat Top"=6, "4 Term B-Harris "=7, "7 Term B-Harris"=8, "Low Sidelobe"=9, "Blackman Nuttall"=11, "Triangle"=30, "Bartlett-Hanning"=31, "Bohman"=32, "Parzen"=33, "Welch"=34, "Kaiser"=60, "Dolph-Chebyshev"=61, "Gaussian"=62] ("window")
        n102 = Index Array(array=w254, index (row)=0) -> (element=w253:i32[])  [unwired: 1 in]
        n103 = Bundle By Name("Y"=w253, "dt"=w252) -> (w251:waveform(i32))  [unwired: 1 in]
        "pdwave" <- w251
        n104 = local read "423 F (Hz)"() -> (w249:i32)
        n105 = local read "532 F (Hz)"() -> (w248:i32)
        n106 = local read "782 F (Hz)"() -> (w247:i32)
        n107 = call-poly <vilib>:"FFT Spectrum (Mag-Phase).vi"("window"=w259, "time signal"=w251) -> ("error out"=w228:errorcluster, "magnitude"=w250:cluster{"f0":dbl, "df":dbl, "magnitude":dbl[]})  [unwired: 5 in, 3 out]
        "pdfft" <- w250
        n108 = call-poly "fftGetMagsPoly.vi"("input cluster"=w250, "422 F (Hz)"=w249, "532 F (Hz)"=w248, "785 F (Hz)"=w247, "unit cal, scu"=w246) -> ("mag422 (mV)"=w241:dbl, "mag532 (mV)"=w240:dbl, "mag785 (mV)"=w239:dbl)  [unwired: 8 in]
        n109 = Bundle("X"=w258, "mag422 (mV)"=w241) -> (w245:cluster{"X":dbl[], "mag422 (mV) ":dbl})  [unwired: 1 in]
        n110 = Bundle("X"=w257, "mag532 (mV)"=w240) -> (w244:cluster{"X":dbl[], "mag532 (mV)":dbl})  [unwired: 1 in]
        n111 = Bundle("X"=w256, "mag785 (mV)"=w239) -> (w243:cluster{"X":dbl[], "mag785 (mV)":dbl})  [unwired: 1 in]
        n112 = call-poly "rollingAverage_multi.vi"("Magnitude Averaging (no. Avgs.)"="Chart Rolling Average", "785nm"=w243, "532nm"=w244, "422nm"=w245) -> ("785nm Data"=w236:T9, "532nm Data"=w237:T10, "422nm Data"=w238:T11)  [unwired: 5 in]
        n113 = call-poly "pdNormalize.vi"("422 Data"=w238, "532 Data"=w237, "785 Data"=w236, "422 PD Cal 3"=w231, "532 PD Cal 3"=w230, "785 PD Cal 3"=w229) -> ("pd ts (raw)"=→"pd ts (raw)":T1, "pd ts"=w235:cluster{dbl, dbl, dbl}, "422 New Array"=w234:dbl[], "532 New Array"=w233:dbl[], "785 New Array"=w232:dbl[])  [unwired: 5 in]
        "pd ts" <- w235
      }
      frame Error {
      }
    }
    n114 = Enqueue Element(queue=w213, element=w210, error in (no error)=w214) -> (queue out=w212:refnum<queue>, error out=w211:errorcluster)  [unwired: 1 in, 1 out]
  }
  n115 = while {
    tunnel: w3 -> [w266]
    tunnel: w2 -> [w265]
    stop <- w272 stop-if-true
    # "Absorption Data Loop (Consummer II)"
    n116 = Dequeue Element(queue=w265) -> (element=w273:cluster{dbl, dbl, dbl}, error out=w271:errorcluster)  [unwired: 2 in, 2 out]
    n117 = Dequeue Element(queue=w266) -> (element=w268:cluster{dbl, dbl, dbl}, error out=w270:errorcluster)  [unwired: 2 in, 2 out]
    n118 = Wait (ms)(milliseconds to wait="save interval (ms)") -> ()  [unwired: 1 out]
    n119 = Merge Errors(w271, w270) -> (w269:errorcluster)
    n120 = case shown="No Error" w269 {
      selector: w269 -> [w306 w311]
      tunnel: w273 -> [w278 _]
      tunnel: [w293 w311] -> w272
      tunnel: w268 -> [w277 _]
      frame No Error {
        w280 = 0.0
        n121 = call-poly "absCalcPlot.vi"("Cell Calibration, mV/mW"="cellcal", "Error In"=w306, "PD Values"="Bkg Values (mV)", "bkg values"=w277, "Mic Values"=w278) -> ("Error Out"=w294:errorcluster, "aae"=→"AAE":dbl, "Time Series"=→"abs ts":cluster{dbl, dbl, dbl}, "Spectrum"=→"Absorption Spectrum":cluster{dbl[], "Best Power Fit":dbl[]}[])  [unwired: 3 in]
        n122 = local read "Elapsed Time (min)"() -> (w283:dbl)
        n123 = local read "pd ts (raw)"() -> (w305:T1)
        n124 = local read "Filtering"() -> (w287:bool)
        n125 = local read "mic ts"() -> (w298:T5)
        n126 = local read "abs ts"() -> (w292:cluster{dbl, dbl, dbl})
        n127 = local read "Calculated Resonance (Hz)"() -> (w288:dbl)
        n128 = Boolean To (0,1)(Boolean=w287) -> (0, 1=w286:i16)
        n129 = Unbundle(w298) -> ("422 Mean"=w297:dbl, "532 Mean"=w296:dbl, "785 Mean"=w295:dbl)
        n130 = Unbundle(w305) -> ("405 Mean"=w299:dbl, "532 Mean"=w300:dbl, "660 Mean"=w301:dbl)
        n131 = Unbundle(w292) -> (w291:dbl, w290:dbl, w289:dbl)
        n132 = To Double Precision Float(number=w286) -> (double precision float=w285:dbl)
        n133 = Format Date/Time String(time format string (%c)="%Y-%m-%d %H:%M:%S\t") -> (date/time string=w302:string)  [unwired: 2 in]
        n134 = Format Into String(format string="%.4e\t%.4e\t%.4e\t%.4e\t%.4e\t%.4e\t%.4e\t%.4e\t%.4e\t%.4e\t%.4e\t%.4e\t%.4e\t%.4e\t%f\t%f\t%.1f", initial string=w302, error in=w294, w297, w296, w295, w280, w299, w300, w301, w280, w280, w291, w290, w289, w280, w280, w288, w285, w283) -> (resulting string=w284:string, error out=w293:errorcluster)
        n135 = local read "PAS Save"() -> (w279:bool)
        n136 = case shown="True" w279 {
          tunnel: w284 -> [_ w308]
          frame False {
          }
          frame True {
            n137 = local read "pas"() -> (w307:path)
            n138 = Build Array(w308) -> (w310:string[])
            n139 = call-poly <vilib>:"Write To Spreadsheet File.vi"("append to file? (new file:F)"=TRUE, "1D data"=w310, "file path (dialog if empty)"=w307) -> ()  [unwired: 5 in, 1 out]
          }
        }
      }
      frame Error {
      }
    }
  }
  n140 = while "Message Processor" {
    shift-left: w64 -> [w325]
    shift-right: [w317] -> w60
    tunnel: w49 -> [w324]
    shift-left: "State Variables" -> [w330]
    shift-right: [w329] -> _
    tunnel: "423 Port" -> [w321]
    tunnel: "532 Port" -> [w320]
    tunnel: "782 Port" -> [w319]
    tunnel: "Teensy Port" -> [w318]
    shift-right: [w315] -> _
    shift-left: _ -> [w314]
    tunnel: w1 -> [w312]
    stop <- w328 stop-if-true
    w322 = 100  # Timeout
    n141 = call "QMH Get Next Message from Queue.vi"("error in (no error)"=w325, "ms timeout (1)"=w322, "queue in"=w324) -> ("error out"=w326:errorcluster, "Next Parameter"=w313:string, "Next Message"=w323:string, "queue out"=w327:refnum<queue>, "Stop QMH"=w328:bool)  [unwired: 3 in]
    n142 = case shown="\"freqset\"" w323 {
      selector: w323 -> [_ w357 _ _ _ _ _ _ _ _ _ _ _ _ _ _ _ _ _ _]
      tunnel: [w353 w358 w371 w381 w440 w463 w495 w502 w508 w514 w520 w528 w535 w542 w562 w569 w593 w605 w623 w634] -> w329
      tunnel: w330 -> [w353 w358 w371 w381 w440 w463 w495 w502 w508 w514 w520 w528 w535 w542 w562 w569 w593 w605 w623 w634]
      tunnel: w327 -> [_ _ _ w374 _ _ _ _ _ _ _ _ _ _ _ _ _ _ w621 w635]
      tunnel: w326 -> [w346 w354 w369 w380 w438 w458 w498 w504 w510 w512 w516 w525 w532 w540 w563 w566 w591 w604 w622 w636]
      tunnel: [w345 w354 w360 w373 w437 w460 w494 w500 w506 w512 w519 w526 w533 w536 w563 w565 w590 w604 w619 w625] -> w317
      tunnel: w321 -> [w343 _ w370 w372 _ _ w497 _ _ _ w521 _ _ w539 _ _ _ _ _ w631]
      tunnel: w320 -> [w342 _ w366 w376 _ _ _ w501 _ _ _ w527 _ w538 _ _ _ _ _ w630]
      tunnel: w319 -> [w341 _ w365 w379 _ _ _ _ w507 _ _ _ w534 w537 _ _ _ _ _ w629]
      tunnel: w318 -> [_ _ w363 w375 w439 w461 _ _ _ _ _ _ _ _ _ w567 w592 _ _ w632]
      tunnel: w313 -> [_ _ _ _ w436 w456 _ _ _ _ w518 w522 w529 _ _ _ w589 w603 _ _]
      tunnel: w312 -> [_ _ _ _ _ _ _ _ _ _ _ _ _ _ _ _ _ w602 _ _]
      frame "", "Wait" {
        # "Update the front panel"
        # "Idle Case - this case is called after a Timeout on the Get Next Message from Queue VI, if no new messages are present on the queue. This case can be used for housekeeping tasks such as updating the UI."
        n143 = Get Date/Time String(want seconds? (F)=TRUE) -> (date string=w352:string, time string=w351:string)  [unwired: 2 in]
        n144 = call "laserDiagnose_III.vi"("405 Port"=w343, "532 Port in"=w342, "660 Port 3"=w341, "error in (no error)"=w346) -> ("Temperatures"=→"Laser Temperatures":T4, "Overtemp"=→"Overtemp":bool, "error out"=w345:errorcluster)  [unwired: 7 in, 2 out]
        n145 = Concatenate Strings(w352, " " ("string"), w351) -> (→"Status":string)
      }
      frame Default {
        # "Call this case if a message is received that is not handled \nby any other case. Typically this is a programming error\nas a result of a typo or unhandled message/missing message handler."
        n146 = Format Into String(format string="DevError: Missing message handler for '%s\" message." ("message"), w357) -> (resulting string=w355:string)  [unwired: 2 in, 1 out]
        n147 = One Button Dialog(message=w355) -> ()  [unwired: 1 in, 1 out]
      }
      frame "Initialize" {
        w367 = u32 115200 ("baud rate (9600)")
        # "Initialize the state variables and user interface\nInitialize serial connections"
        n148 = call-poly "VISA Configure Serial Port"("VISA resource name"=w370, "baud rate (9600)"=w367, "error in (no error)"=w369) -> ("error out"=w368:errorcluster)  [unwired: 11 in, 1 out]
        n149 = call-poly "VISA Configure Serial Port"("VISA resource name"=w366, "baud rate (9600)"=w367, "error in (no error)"=w368) -> ("error out"=w364:errorcluster)  [unwired: 11 in, 1 out]
        n150 = call-poly "VISA Configure Serial Port"("VISA resource name"=w365, "baud rate (9600)"=w367, "error in (no error)"=w364) -> ("error out"=w362:errorcluster)  [unwired: 11 in, 1 out]
        n151 = call-poly "VISA Configure Serial Port"("VISA resource name"=w363, "error in (no error)"=w362) -> ("VISA resource name out"=w361:refnum<visa-resource-name>, "error out"=w359:errorcluster)  [unwired: 12 in]
        n152 = property class="Instr" props=["Baud"](reference=w361, error in=w359) -> (error out=w360:errorcluster)  [unwired: 2 out]
      }
      frame "sweep" {
        # "Perform a frequency sweep and calculate the resonance frequency"
        n153 = stacked-sequence {
          seq-local: [_ w394 _ _] -> [_ _ w422 _]
          tunnel: w380 -> [_ w388 _ _]
          tunnel: "Data End Frequency (Hz)" -> [_ w391 w416 _]
          tunnel: "Data Start Frequency (Hz)" -> [_ w390 w415 _]
          tunnel: w379 -> [w384 _ _ w428]
          tunnel: w376 -> [w382 _ _ w427]
          tunnel: w375 -> [_ w389 _ _]
          tunnel: w374 -> [_ _ _ w433]
          tunnel: [_ _ _ w429] -> w373
          tunnel: w372 -> [_ _ _ _]
          frame #0 {
            w387 = FALSE
            # "Turn red and green lasers off for scan."
            n154 = call "laserOnOff.vi"("Emission (F = OFF)"=w387, "VISA Refnum in"=w382) -> ("error out"=w386:errorcluster)  [unwired: 7 in, 2 out]
            n155 = Wait (ms)(milliseconds to wait=u32 5000) -> ()  [unwired: 1 out]
            n156 = local write "Status"("Conducting Frequency Sweep" ("Status")) -> ()
            n157 = call "laserOnOff.vi"("error in (no error)"=w386, "Emission (F = OFF)"=w387, "VISA Refnum in"=w384) -> ()  [unwired: 6 in, 3 out]
          }
          frame #1 {
            n158 = Subtract(x=w391, y=w390) -> (x-y=w392:i32)
            n159 = for {
              N: w392 -> [w398]
              tunnel: [w403] -> w394 mode=indexing
              tunnel: w390 -> [w402]
              tunnel: w391 -> [w401]
              tunnel: w388 -> [_]
              i -> [w395]
              # "Get microphone data."
              # "Listen for N*2000\n seconds"
              n160 = Increment(x=w395) -> (x+1=w396:i32)
              n161 = Divide(x=w396, y=w398) -> (x/y=→"sweep progress":dbl)
              n162 = local read "micfft"() -> (w400:cluster{"f0":dbl, "df":dbl, "magnitude":dbl[]})
              n163 = Unbundle By Name(w400) -> ("magnitude"=w399:dbl[])
              n164 = Wait (ms)(milliseconds to wait=u32 2000) -> ()  [unwired: 1 out]
              n165 = call "fftGetMax.vi"("End Frequency (Hz)"=w401, "Start Frequency (Hz)"=w402, "Magnitudes"=w399) -> ("max value"=w403:dbl)  [unwired: 8 in]
            }
            n166 = case shown="False" TRUE ("sweep?") {
              tunnel: w390 -> [_ w410]
              tunnel: w391 -> [_ w409]
              tunnel: w389 -> [_ w408]
              tunnel: [w405 w407] -> _
              tunnel: w388 -> [w405 w406]
              frame False {
              }
              frame True {
                # "Scan laser freq.\nwith Teensy"
                n167 = call "teensySweepFreq.vi"("error in (no error)"=w406, "end f, Hz (1385)"=w409, "start f, Hz (1355)"=w410, "VISA Refnum in"=w408) -> ("error out"=w407:errorcluster)  [unwired: 7 in]
              }
            }
          }
          frame #2 {
            # "Calculate resonance frequency;\ndisplay and save scan."
            n168 = Wait (ms)(milliseconds to wait=u32 5000) -> ()  [unwired: 1 out]
            n169 = local read "PAS Save"() -> (w411:bool)
            n170 = To Double Precision Float(number=w416) -> (double precision float=w413:dbl)
            n171 = To Double Precision Float(number=w415) -> (double precision float=w414:dbl)
            n172 = call "resCalc.vi"("Frequency Sweep"=w422, "Start F, Hz (1355)"=w415) -> ("F-res, Hz"=w420:dbl, "Frequency Scan"=w412:cluster{i32[], "Best Gaussian Fit":dbl[]}[])  [unwired: 8 in]
            "freqscan" <- w412
            n173 = In Range and Coerce(upper limit=w413, x=w420, lower limit=w414) -> (In Range?=w419:bool)  [unwired: 1 out]
            n174 = case shown="True" w411 {
              tunnel: w412 -> [_ w426]
              tunnel: w420 -> [_ w425]
              frame False {
              }
              frame True {
                n175 = local read "sweeps"() -> (w424:path)
                n176 = call "saveFreqSweep.vi"("f-res, Hz"=w425, "Frequency Scan"=w426, "file path (dialog if empty)"=w424) -> ()  [unwired: 9 in]
              }
            }
            n177 = And(x=w419, y=TRUE ("check freqs?")) -> (x .and. y?=w417:bool)
            n178 = case shown="True" w417 {
              tunnel: w420 -> [_ w423]
              frame False {
              }
              frame True {
                n179 = property on="Calculated Resonance (Hz)" class="DigNum (strict)"("Val(Sgnl)"=w423) -> ()  [unwired: 2 in, 2 out]
                "Calculated Resonance (Hz)" <- w423
              }
            }
          }
          frame #3 {
            w434 = TRUE
            # "Turn red and green lasers back on."
            n180 = call "laserOnOff.vi"("Emission (F = OFF)"=w434, "VISA Refnum in"=w427) -> ("error out"=w435:errorcluster)  [unwired: 7 in, 2 out]
            n181 = call "laserOnOff.vi"("error in (no error)"=w435, "Emission (F = OFF)"=w434, "VISA Refnum in"=w428) -> ("error out"=w430:errorcluster)  [unwired: 6 in, 2 out]
            n182 = call-poly "QMH Add Message to Queue.vi"("error in (no error)"=w430, "Parameter"="532 F (Hz)", "Message"="freqset", "queue in"=w433) -> ("error out"=w429:errorcluster)  [unwired: 6 in, 1 out]
          }
        }
      }
      frame "freqset" {
        # "Set the frequency of the Teensy's modulation\nsignal for single laser (if single frequency is changed)."
        # "Set the laser frequency.  Case for \"red\", \"blue\", or \"green\"."
        n183 = case shown="\"782 F (Hz)\"" w436 {
          tunnel: w438 -> [w445 w450 w455]
          tunnel: [w444 w449 w454] -> w437
          tunnel: w439 -> [w441 w446 w452]
          frame "405 F (Hz) ", Default {
            w443 = u16 0 items=["blue", "green", "red"] ("laser")
            n184 = call "freqSet.vi"("error in (no error)"=w445, "laser"=w443, "Freq, Hz (1370)"="423 F (Hz)", "Teensy Port"=w441) -> ("error out"=w444:errorcluster)  [unwired: 6 in, 1 out]
          }
          frame "532 F (Hz)" {
            w448 = u16 1 items=["blue", "green", "red"] ("laser")
            n185 = call "freqSet.vi"("error in (no error)"=w450, "laser"=w448, "Freq, Hz (1370)"="532 F (Hz)", "Teensy Port"=w446) -> ("error out"=w449:errorcluster)  [unwired: 6 in, 1 out]
          }
          frame "782 F (Hz)" {
            w451 = u16 2 items=["blue", "green", "red", "ir"] ("laser")
            n186 = call "freqSet.vi"("error in (no error)"=w455, "laser"=w451, "Freq, Hz (1370)"="782 F (Hz)", "Teensy Port"=w452) -> ("error out"=w454:errorcluster)  [unwired: 6 in, 1 out]
          }
        }
      }
      frame "setfreqs" {
        # "Set the frequency of the Teensy's modulation\nsignal for all lasers at once."
        # "Set laser frequencies to resonance frequency calculated in sweep."
        n187 = Scan From String(input string=w456, error in=w458) -> (error out=w457:errorcluster, output 1=w459:dbl)  [unwired: 3 in, 2 out]
        n188 = for {
          N: 3 -> [_]
          tunnel: [w469] -> w460
          tunnel: w457 -> [w468]
          tunnel: w461 -> [w465]
          tunnel: w459 -> [w467]
          i -> [w466]
          n189 = flat-sequence {
            tunnel: w465 -> [w470]
            tunnel: [w470] -> w464
            frame #0 {
              n190 = Wait (ms)(milliseconds to wait=u32 1000) -> ()  [unwired: 1 out]
            }
          }
          n191 = case shown="0" w466 {
            tunnel: [w477 w485 w493] -> w469
            tunnel: w468 -> [w475 w482 w490]
            tunnel: w464 -> [w474 w481 w489]
            tunnel: w467 -> [w472 w478 w486]
            frame 0 {
              w476 = u16 2 items=["blue", "green", "red"] ("laser")
              n192 = To Long Integer(number=w472) -> (32bit integer=w473:i32)
              n193 = local write "782 F (Hz)"(w473) -> ()
              n194 = call "freqSet.vi"("error in (no error)"=w475, "laser"=w476, "Freq, Hz (1370)"=w473, "Teensy Port"=w474) -> ("error out"=w477:errorcluster)  [unwired: 6 in, 1 out]
            }
            frame 1, Default {
              w484 = u16 1 items=["blue", "green", "red"] ("laser")
              n195 = Add(x=w478, y=2.0) -> (x+y=w480:dbl)
              n196 = To Long Integer(number=w480) -> (32bit integer=w479:i32)
              n197 = call "freqSet.vi"("error in (no error)"=w482, "laser"=w484, "Freq, Hz (1370)"=w479, "Teensy Port"=w481) -> ("error out"=w485:errorcluster)  [unwired: 6 in, 1 out]
              n198 = local write "532 F (Hz)"(w479) -> ()
            }
            frame 2 {
              w492 = u16 0 items=["blue", "green", "red"] ("laser")
              n199 = Subtract(x=w486, y=2.0) -> (x-y=w488:dbl)
              n200 = To Long Integer(number=w488) -> (32bit integer=w487:i32)
              n201 = call "freqSet.vi"("error in (no error)"=w490, "laser"=w492, "Freq, Hz (1370)"=w487, "Teensy Port"=w489) -> ("error out"=w493:errorcluster)  [unwired: 6 in, 1 out]
              n202 = local write "423 F (Hz)"(w487) -> ()
            }
          }
        }
      }
      frame "405 emit" {
        # "Turn laser on or off"
        n203 = call "laserOnOff.vi"("error in (no error)"=w498, "Emission (F = OFF)"="423 Emission", "Power, mW (100)"="423 Power (mW)", "VISA Refnum in"=w497) -> ("error out"=w494:errorcluster)  [unwired: 5 in, 2 out]
      }
      frame "532 emit" {
        # "Turn laser on or off"
        n204 = call "laserOnOff.vi"("error in (no error)"=w504, "Emission (F = OFF)"="532 Emission", "Power, mW (100)"="532 Power (mW)", "VISA Refnum in"=w501) -> ("error out"=w500:errorcluster)  [unwired: 5 in, 2 out]
      }
      frame "660 emit" {
        # "Turn laser on or off"
        n205 = call "laserOnOff.vi"("error in (no error)"=w510, "Emission (F = OFF)"="782 Emission", "Power, mW (100)"="782 Power (mW)", "VISA Refnum in"=w507) -> ("error out"=w506:errorcluster)  [unwired: 5 in, 2 out]
      }
      frame "emit" {
        # "Turn on all lasers."
        n206 = local write "423 Emission"("All Emit") -> ()
        n207 = local write "532 Emission"("All Emit") -> ()
        n208 = local write "782 Emission"("All Emit") -> ()
      }
      frame "405 Power" {
        # "Set laser power"
        n209 = Scan From String(input string=w518, error in=w516) -> (error out=w515:errorcluster, output 1=w517:dbl)  [unwired: 3 in, 2 out]
        n210 = call "laserSetPower.vi"("error in (no error)"=w515, "Laser Power (mW)"=w517, "VISA Refnum in"=w521) -> ("error out"=w519:errorcluster)  [unwired: 7 in, 1 out]
      }
      frame "532 Power" {
        n211 = Scan From String(input string=w522, error in=w525) -> (error out=w524:errorcluster, output 1=w523:dbl)  [unwired: 3 in, 2 out]
        n212 = call "laserSetPower.vi"("error in (no error)"=w524, "Laser Power (mW)"=w523, "VISA Refnum in"=w527) -> ("error out"=w526:errorcluster)  [unwired: 7 in, 1 out]
      }
      frame "782 Power" {
        n213 = Scan From String(input string=w529, error in=w532) -> (error out=w531:errorcluster, output 1=w530:dbl)  [unwired: 3 in, 2 out]
        n214 = call "laserSetPower.vi"("error in (no error)"=w531, "Laser Power (mW)"=w530, "VISA Refnum in"=w534) -> ("error out"=w533:errorcluster)  [unwired: 7 in, 1 out]
      }
      frame "align" {
        # "Set power of all lasers to 5 mW for alignment"
        n215 = case shown="True" "Alignment Mode" {
          tunnel: w540 -> [w550 w560]
          tunnel: w539 -> [w549 w559]
          tunnel: w538 -> [w548 w558]
          tunnel: w537 -> [w547 w557]
          tunnel: [w544 w554] -> w536
          frame True {
            w543 = 5.0 ("Laser Power (mW)")
            n216 = call "laserSetPower.vi"("error in (no error)"=w550, "Laser Power (mW)"=w543, "VISA Refnum in"=w549) -> ("error out"=w546:errorcluster)  [unwired: 7 in, 1 out]
            n217 = call "laserSetPower.vi"("error in (no error)"=w546, "Laser Power (mW)"=w543, "VISA Refnum in"=w548) -> ("error out"=w545:errorcluster)  [unwired: 7 in, 1 out]
            n218 = call "laserSetPower.vi"("error in (no error)"=w545, "Laser Power (mW)"=w543, "VISA Refnum in"=w547) -> ("error out"=w544:errorcluster)  [unwired: 7 in, 1 out]
          }
          frame False, Default {
            n219 = local read "423 Power (mW)"() -> (w553:dbl)
            n220 = local read "532 Power (mW)"() -> (w552:dbl)
            n221 = local read "782 Power (mW)"() -> (w551:dbl)
            n222 = call "laserSetPower.vi"("error in (no error)"=w560, "Laser Power (mW)"=w553, "VISA Refnum in"=w559) -> ("error out"=w556:errorcluster)  [unwired: 7 in, 1 out]
            n223 = call "laserSetPower.vi"("error in (no error)"=w556, "Laser Power (mW)"=w552, "VISA Refnum in"=w558) -> ("error out"=w555:errorcluster)  [unwired: 7 in, 1 out]
            n224 = call "laserSetPower.vi"("error in (no error)"=w555, "Laser Power (mW)"=w551, "VISA Refnum in"=w557) -> ("error out"=w554:errorcluster)  [unwired: 7 in, 1 out]
          }
        }
      }
      frame "background" {
        n225 = local read "mic ts"() -> (w561:T5)
        n226 = local write "Bkg Values (mV)"(w561) -> ()
      }
      frame "filter" {
        n227 = local read "Filtering"() -> (w568:bool)
        n228 = case shown="True" w568 {
          tunnel: w567 -> [w572 w581]
          tunnel: w566 -> [w571 w579]
          tunnel: [w570 w580] -> w565
          frame False {
            n229 = Multiply(x="Filter Length (min)", y=60.0) -> (x*y=w575:dbl)
            n230 = local write "Time Target (s)"(w575) -> ()
            n231 = VISA Write(VISA resource name=w572, write buffer="v.1", error in (no error)=w571) -> (error out=w570:errorcluster)  [unwired: 2 out]
            "Filtering" <- TRUE
          }
          frame True {
            n232 = flat-sequence {
              tunnel: w579 -> [w587]
              tunnel: [w587] -> w578
              frame #0 {
                n233 = local read "mic ts"() -> (w588:T5)
                n234 = local write "Bkg Values (mV)"(w588) -> ()
              }
            }
            n235 = local write "Filtering"(FALSE) -> ()
            n236 = VISA Write(VISA resource name=w581, write buffer="v.0", error in (no error)=w578) -> (error out=w580:errorcluster)  [unwired: 2 out]
            n237 = Multiply(x="Sample Length (min)", y=60.0) -> (x*y=w583:dbl)
            n238 = local write "Time Target (s)"(w583) -> ()
          }
        }
        n239 = Wait (ms)(milliseconds to wait=u32 500) -> ()  [unwired: 1 out]
      }
      frame "filterswitch" {
        n240 = case shown="\"TRUE\"" w589 {
          tunnel: w592 -> [w596 w601]
          tunnel: w591 -> [w595 w600]
          tunnel: [w594 w599] -> w590
          frame "FALSE", Default {
            n241 = VISA Write(VISA resource name=w596, write buffer="v.0", error in (no error)=w595) -> (error out=w594:errorcluster)  [unwired: 2 out]
          }
          frame "TRUE" {
            n242 = VISA Write(VISA resource name=w601, write buffer="v.1", error in (no error)=w600) -> (error out=w599:errorcluster)  [unwired: 2 out]
          }
        }
      }
      frame "namefiles" {
        n243 = case shown="\"TRUE\"" w603 {
          tunnel: w602 -> [_ w607]
          frame "FALSE", Default {
            n244 = local write "PAS Save"(FALSE ("PAS Save")) -> ()
          }
          frame "TRUE" {
            n245 = flat-sequence {
              tunnel: [w612] -> w610
              tunnel: [w614] -> w609
              tunnel: w610 -> [w614]
              tunnel: w609 -> [w616]
              tunnel: w608 -> [w615]
              frame #0 {
                n246 = call "saveSetDirectory.vi"() -> ("pas"=w612:path, "sweeps"=→"sweeps":path)  [unwired: 11 in, 3 out]
                "pas" <- w612
              }
              frame #1 {
                "PAS Save" <- TRUE ("PAS Save")
              }
              frame #2 {
                n247 = call-poly <vilib>:"Write To Spreadsheet File.vi"("append to file? (new file:F)"=TRUE, "2D data"=w615, "file path (dialog if empty)"=w616) -> ()  [unwired: 5 in, 1 out]
              }
            }
            n248 = Build Array(w607) -> (w608:string[][])
          }
        }
      }
      frame "Error" {
        (unwired) errorcluster {"status"=FALSE, "code"=0, "source"=""} ("error out")
        # "Proceed to Exit - remove if this is\nnot appropriate for the General Error case"
        # "General Error Case - this case is called if an error is passed using the error cluster below. Typically most new errors should be handed in each individual case and not passed in the rror cluster. If necessary a custom error handler case should be added and called from other cases."
        n249 = call <vilib>:"Simple Error Handler.vi"("error in (no error)"=w622) -> ("error out"=w618:errorcluster)  [unwired: 4 in, 4 out]
        n250 = call-poly "QMH Add Message to Queue.vi"("error in (no error)"=w618, "Message"="Exit", "queue in"=w621) -> ("error out"=w619:errorcluster)  [unwired: 7 in, 1 out]
      }
      frame "Exit" {
        # "Perform cleanup tasks: Close serial connections and clear front panel."
        n251 = call "QMH Destroy Queue.vi"("error in (no error)"=w636, "queue in"=w635) -> ("error out"=w628:errorcluster)  [unwired: 7 in, 2 out]
        n252 = for {
          N: 3 -> [_]
          tunnel: w631 -> [w643]
          tunnel: w630 -> [w641]
          tunnel: w629 -> [w640]
          tunnel: w628 -> [w639]
          tunnel: FALSE -> [w638]
          tunnel: [w637] -> w624
          i -> [w642]
          # "Close laser serial connections."
          n253 = case shown="0, Default" w642 {
            tunnel: [w650 w655 w660] -> w645
            tunnel: [w649 w654 w659] -> w644
            tunnel: w643 -> [w648 _ _]
            tunnel: w641 -> [_ w653 _]
            tunnel: w640 -> [_ _ w657]
            tunnel: w639 -> [w647 w652 w658]
            tunnel: w638 -> [w646 w651 w656]
            frame 0, Default {
              n254 = call "laserOnOff.vi"("error in (no error)"=w647, "Emission (F = OFF)"=w646, "VISA Refnum in"=w648) -> ("error out"=w650:errorcluster, "VISA Refnum out"=w649:refnum<visa-resource-name>)  [unwired: 6 in, 1 out]
              n255 = local write "423 Emission"(w646) -> ()
            }
            frame 1 {
              n256 = call "laserOnOff.vi"("error in (no error)"=w652, "Emission (F = OFF)"=w651, "VISA Refnum in"=w653) -> ("error out"=w655:errorcluster, "VISA Refnum out"=w654:refnum<visa-resource-name>)  [unwired: 6 in, 1 out]
              n257 = local write "532 Emission"(w651) -> ()
            }
            frame 2 {
              n258 = call "laserOnOff.vi"("error in (no error)"=w658, "Emission (F = OFF)"=w656, "VISA Refnum in"=w657) -> ("error out"=w660:errorcluster, "VISA Refnum out"=w659:refnum<visa-resource-name>)  [unwired: 6 in, 1 out]
              n259 = local write "782 Emission"(w656) -> ()
              n260 = local write "All Emit"(w656) -> ()
            }
          }
          n261 = VISA Close(VISA resource name=w644, error in (no error)=w645) -> (error out=w637:errorcluster)
        }
        n262 = local write "Status"("" ("Status")) -> ()
        n263 = VISA Close(VISA resource name=w632, error in (no error)=w624) -> (error out=w625:errorcluster)
      }
    }
    n264 = case shown="True" "Auto Filter" {
      tunnel: [w331 w333] -> w315
      tunnel: w314 -> [w331 w332]
      frame False {
      }
      frame True {
        # "This is the timer for the filtering routine."
        n265 = call "Elapsed Time"("Time Target (s)"="Time Target (s)", "Auto Reset"=TRUE, "error in (no error)"=w332) -> ("Elapsed Time (s)"=w336:dbl, "Time has Elapsed"=w338:bool, "error out"=w337:errorcluster)  [unwired: 9 in, 5 out]
        "Time has Elapsed" <- w338
        n266 = Divide(x=w336, y=60.0) -> (x/y=→"Elapsed Time (min)":dbl)
        n267 = property on="Time has Elapsed" class="Bool (strict)"(error in=w337, "Val(Sgnl)"=w338) -> (error out=w333:errorcluster)  [unwired: 1 in, 1 out]
      }
    }
  }
  n268 = Release Queue(queue=w10, error in (no error)=w9) -> ()  [unwired: 1 in, 3 out]
  n269 = Merge Errors(w60, w50) -> (w59:errorcluster)
  n270 = Release Queue(queue=w7, error in (no error)=w6) -> ()  [unwired: 1 in, 3 out]
  n271 = call <vilib>:"Simple Error Handler.vi"("error in (no error)"=w59) -> ("error out"=w58:errorcluster)  [unwired: 4 in, 4 out]
  n272 = flat-sequence {
    tunnel: w58 -> [w661]
    tunnel: [w661] -> w57
    frame #0 {
      n273 = local write "Exit"(FALSE) -> ()
    }
  }
  "Error Console" <- w57
